vi "TCP Get interlock status.vi"(8 "error in (no error)":errorcluster) -> ()   [LabVIEW 2020]
uses:
  Shared/MySQL/Preset Query Enum.ctl
  Interlock status global variable.vi
panel:
  out "Boolean":bool
  out "loop error":errorcluster
  in  "exit loop 2":bool
  out "port":u16
  out "address":string="192.168.14.14"
  out "No error":errorcluster
  in  "exit loop":bool
  out "data out":string
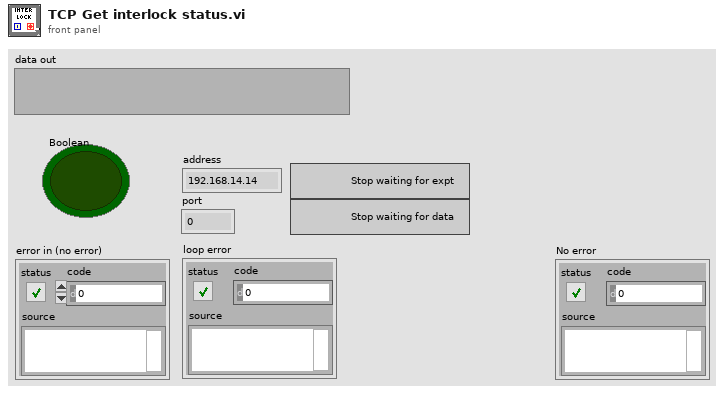
[diagram p1: front panel]
types:
  T1 = typedef "Preset Query Enum.ctl" = enum16{"Get Locations", "Get all IPs and MACs", "Get classes", "Get expt variables to set at scanstart for particular device", "Get expt devices and variables with start values", "Get expt devices and variables (with data to get)", "Get expt devices with data to get", "Get Expt devices and GUIs", "Get all devices basic properties", "Get Virtual Devices Core Info", "Get Expt names", "Get experiment basic properties", "Get experiment alarm variables", "Get MC Ports", "Get device network comm port", "Get devicetype lvclass path", "Get basic device properties", "Get Init Order", "Get all setable variables of a device", "Get device variable aliases", "Get force values of all settable variables", "Get all variables of a devicetype", "Get all variables of a device", "Get plotter details", "Get Saved Scans", "Get Scan Info", "GetGeneralGUIs", "Get expt for plotter", "Get plotter IDs from expt", "Get all devices", "Get all Virtual Devices", "Get all aliases", "Get variable and device info for Virtual Device", "GetItemLocatorIP", "Get IPs for GUIs", "Get DeviceType from Device", "GetLocalPortRange", "GetDevicePresetVariables", "Get Device Configuration", "GetAllPresetNames", "GetAllConfigurationNames", "GetPresetDeviceNames", "GetDeviceAliases", "GetDevicesOfClass"}
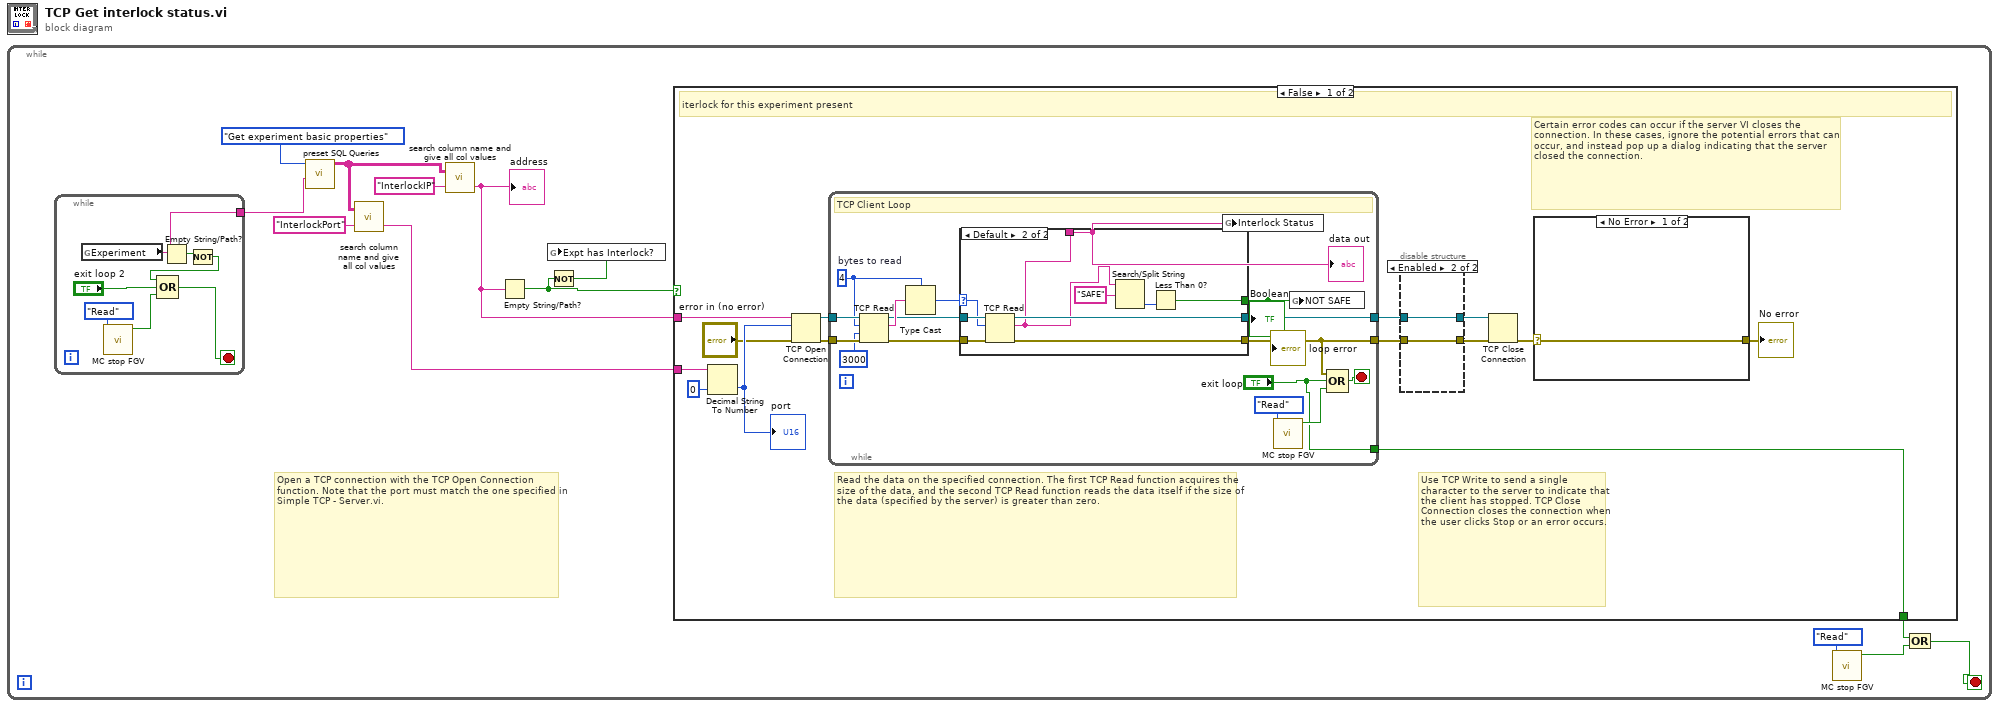
[diagram p0: block diagram]
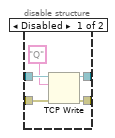
[diagram p2: hidden frame]
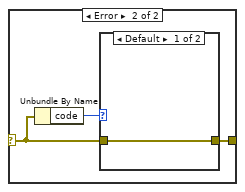
[diagram p3: hidden frame]
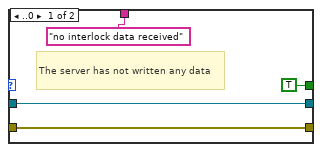
[diagram p5: hidden frame]
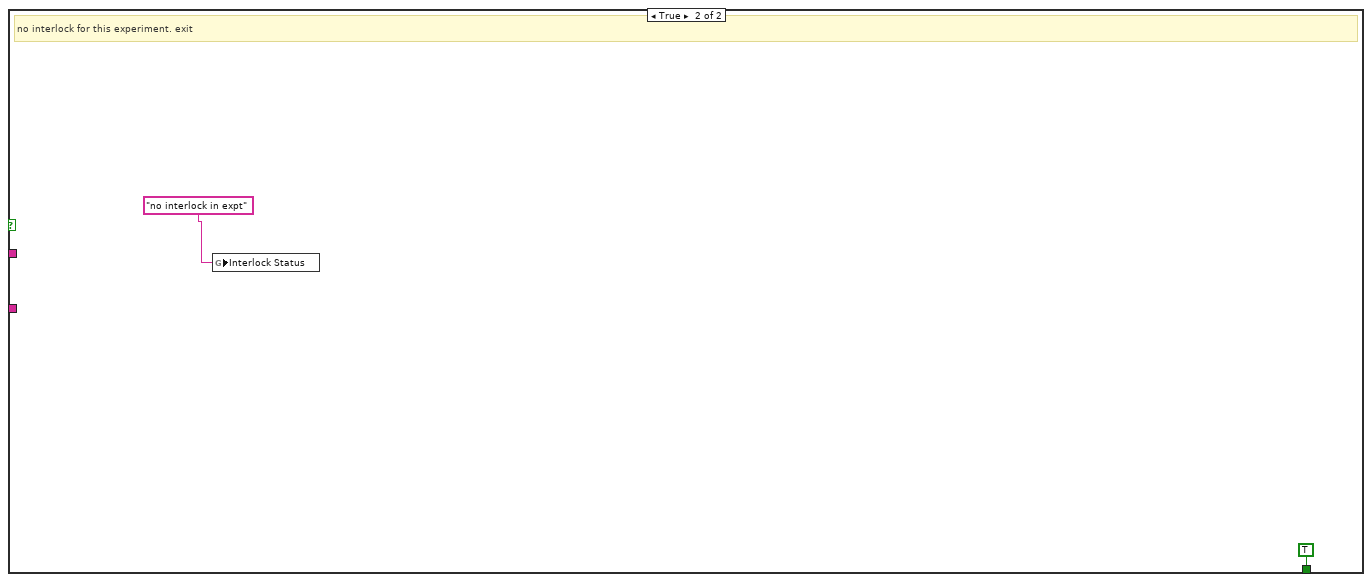
[diagram p6: hidden frame]
diagram:
  n1 = while {
    stop <- w10 stop-if-true
    # "Open a TCP connection with the TCP Open Connection function. Note that the port must match the one specified in Simple TCP - Server.vi."
    n2 = while {
      tunnel: [w72] -> w4
      stop <- w75 stop-if-true
      n3 = global read "Interlock status global variable.vi" "Experiment"() -> (w72:string)
      n4 = call "MC stop FGV.vi"("Function"=enum16{"Read", "Write", "Clear"}."Read") -> ("Stop out"=w77:bool)  [unwired: 9 in, 1 out]
      n5 = Empty String/Path?(string/path=w72) -> (empty?=w74:bool)
      n6 = Not(x=w74) -> (.not. x?=w73:bool)
      n7 = Compound Arithmetic op=OR(w73, "exit loop 2", w77) -> (w75:bool)
    }
    n8 = call "preset SQL Queries.vi"("Expt name / MCIP/ Variable/Preset Name"=w4, "Preset Query"=Preset_Query_Enum."Get experiment basic properties") -> ("data"=w6:string[][])  [unwired: 7 in, 2 out]
    n9 = call "search column name and give all col values.vi"("column name to get"="InterlockPort", "input 2d array"=w6) -> ("First value"=w5:string)  [unwired: 1 out]
    n10 = call "search column name and give all col values.vi"("column name to get"="InterlockIP", "input 2d array"=w6) -> ("First value"=w3:string)  [unwired: 1 out]
    "address" <- w3
    n11 = Empty String/Path?(string/path=w3) -> (empty?=w1:bool)
    n12 = Not(x=w1) -> (.not. x?=w2:bool)
    n13 = global write "Interlock status global variable.vi" "Expt has Interlock?"(w2) -> ()
    n14 = case shown="False" w1 {
      tunnel: [w19 TRUE ("exit loop")] -> w12
      tunnel: w5 -> [w18 _]
      tunnel: w3 -> [w14 _]
      frame False {
        # "Certain error codes can occur if the server VI closes the connection. In these cases, ignore the potential errors that can occur, and instead pop up a dialog indicating that the server closed the connection."
        # "Use TCP Write to send a single character to the server to indicate that the client has stopped. TCP Close Connection closes the connection when the user clicks Stop or an error occurs."
        # "Read the data on the specified connection. The first TCP Read function acquires the size of the data, and the second TCP Read function reads the data itself if the size of the data (specified by the server) is greater than zero."
        # "iterlock for this experiment present"
        n15 = Decimal String To Number(string=w18, default (0L)=u16 0 ("default (0 I32)")) -> (number=w17:u16)  [unwired: 1 in, 1 out]
        "port" <- w17
        n16 = TCP Open Connection(address=w14, remote port or service name=w17, error in (no error)="error in (no error)") -> (connection ID=w27:refnum<k5>, error out=w26:errorcluster)  [unwired: 2 in]
        n17 = while {
          tunnel: w26 -> [w52]
          tunnel: w27 -> [w53]
          tunnel: [w49] -> w24
          tunnel: [w48] -> w22
          tunnel: ["exit loop"] -> w19
          stop <- w50 stop-if-true
          w51 = 4  # bytes to read
          # "TCP Client Loop"
          n18 = TCP Read(connection ID=w53, bytes to read=w51, error in (no error)=w52, 9:3000 ("timeout ms (25000)")) -> (connection ID out=w55:refnum<k5>, data out=w56:string, error out=w54:errorcluster)  [unwired: 1 in]
          n19 = Type Cast(type=w51, x=w56) -> (*(type *) &x=w47:i32)
          n20 = case shown="Default" w47 {
            selector: w47 -> [_ w65]
            tunnel: w55 -> [w60 w69]
            tunnel: w54 -> [w59 w68]
            tunnel: [w60 w67] -> w49
            tunnel: [w59 w66] -> w48
            tunnel: ["no interlock data received" ("data out") w62] -> w42
            tunnel: [TRUE w61] -> w41
            frame ..0 {
              # "The server has not written any data"
            }
            frame Default {
              n21 = TCP Read(connection ID=w69, bytes to read=w65, error in (no error)=w68) -> (connection ID out=w67:refnum<k5>, data out=w62:string, error out=w66:errorcluster)  [unwired: 2 in]
              n22 = Search/Split String(string=w62, search string/char (-)="SAFE") -> (offset of match=w64:i32)  [unwired: 1 in, 2 out]
              n23 = Less Than 0?(x=w64) -> (x < 0?=w61:bool)
            }
          }
          "data out" <- w42
          "loop error" <- w48
          "Boolean" <- w41
          n24 = global write "Interlock status global variable.vi" "Interlock Status"(w42) -> ()
          n25 = call "MC stop FGV.vi"("Function"=enum16{"Read", "Write", "Clear"}."Read") -> ("Stop out"=w44:bool)  [unwired: 9 in, 1 out]
          n26 = global write "Interlock status global variable.vi" "NOT SAFE"(w41) -> ()
          n27 = Compound Arithmetic op=OR(w48, "exit loop", w44) -> (w50:bool)
        }
        n28 = disable-structure shown="Enabled" {
          disable-tunnel: [w32 w34] -> w25
          disable-tunnel: w24 -> [w31 w34]
          disable-tunnel: [w30 w33] -> w23
          disable-tunnel: w22 -> [w29 w33]
          frame Disabled {
            n29 = TCP Write(connection ID=w31, data in="Q", error in (no error)=w29) -> (connection ID out=w32:refnum<k5>, error out=w30:errorcluster)  [unwired: 2 out]
          }
          frame Enabled {
          }
        }
        n30 = TCP Close Connection(connection ID=w25, error in (no error)=w23) -> (error out=w21:errorcluster)  [unwired: 1 in, 1 out]
        n31 = case shown="No Error" w21 {
          selector: w21 -> [w35 w37]
          tunnel: [w35 w36] -> w20
          frame No Error {
          }
          frame Error {
            n32 = Unbundle By Name(w37) -> ("code"=w38:i32)
            n33 = case shown="Default" w38 {
              tunnel: w37 -> [w39 w40]
              tunnel: [w39 w40] -> w36
              frame Default {
              }
              frame 62, 64, 66 {
              }
            }
          }
        }
        "No error" <- w20
      }
      frame True {
        # "no interlock for this experiment. exit"
        n34 = global write "Interlock status global variable.vi" "Interlock Status"("no interlock in expt") -> ()
      }
    }
    n35 = call "MC stop FGV.vi"("Function"=enum16{"Read", "Write", "Clear"}."Read") -> ("Stop out"=w11:bool)  [unwired: 9 in, 1 out]
    n36 = Compound Arithmetic op=OR(w12, w11) -> (w10:bool)
  }
